vi "GageAcquire.vi"() -> ()   [LabVIEW 2015]
panel:
  in  "Force Capture":bool
  in  "Trigger":T1={"Slope"=0, "Level"=0, "Source"=0, "External Range"=2000, "External Coupling"=0, "External"=FALSE, "Disable"=FALSE, "External Impedance"=1} {"External Impedance" items=["50 Ohm", "HiZ"]; "External Coupling" items=["DC", "AC"]; "External Range" min=2000 max=10000 step=8000; "Slope" items=["Rising", "Falling"]; "Level" min=-100 max=100; "Source" min=0 max=64 step=1}
  in  "Channels":T2(array[cluster])=[{"Coupling"=0, "Differential Input"=FALSE, "Direct-to-ADC"=FALSE, "Range"=2000, "Impedance"=50, "DC Offset"=0, "Filter"=0}] {"Impedance" min=50 max=1000000 step=999950; "Coupling" items=["DC", "AC"]}
  in  "Acquisition":T3={"Sample Rate"=100000000.0, "Clock mode"=enum."Internal", "Mode"=0, "Depth"=8192.0, "Segment Size"=8192.0, "Trigger Timeout"=1000000.0, "Trigger Holdoff"=0.0, "Trigger Delay"=0.0} {"Segment Size" min=256.0 step=128.0; "Trigger Holdoff" min=0.0 step=128.0; "Trigger Delay" min=0.0 step=128.0; "Depth" min=256.0 step=128.0; "Mode" items=["Single", "Dual", "Quad", "Octal"]}
  in  "Continuous":bool
  out "Progress":string
  in  "stop":bool
  out "Waveform Graph":cluster{dbl, dbl, "Data in Volts":dbl[][]}(graph)
  out "System Name":string
  out "Sample Bits":i32
  out "Trigger Count":i32
  out "Channel Count":i32
  out "Board Count":i32
  out "System Count":i32
  in  "Points":u32=4096
  in  "Start":dbl
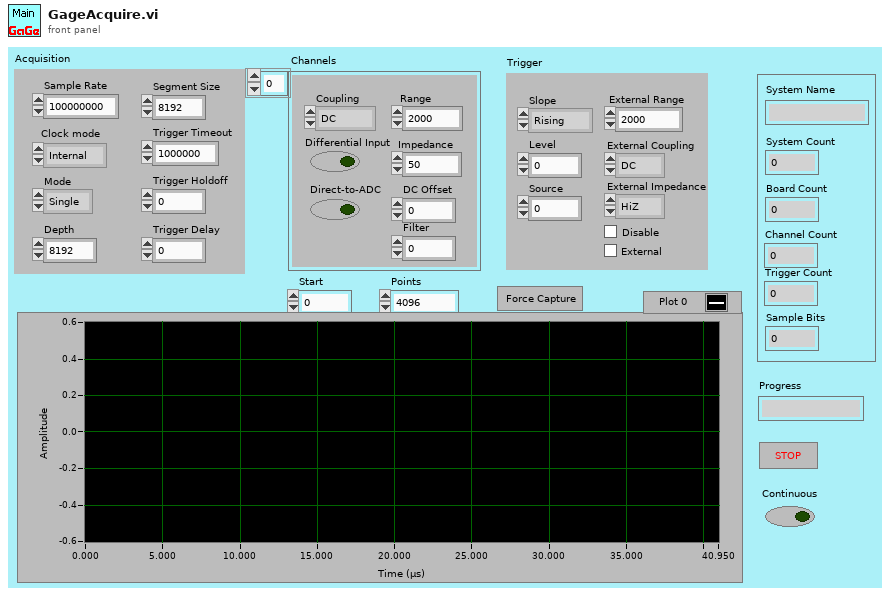
[diagram p1: front panel]
types:
  T1 = cluster{"Slope":u16, "Level":i32, "Source":i32, "External Range":u32, "External Coupling":u16, "External":bool, "Disable":bool, "External Impedance":u16}
  T2 = cluster{"Coupling":u16, "Differential Input":bool, "Direct-to-ADC":bool, "Range":u32, "Impedance":u32, "DC Offset":i32, "Filter":i32}[]
  T3 = cluster{"Sample Rate":dbl, "Clock mode":enum16{"Internal", "External", "Reference"}, "Mode":u16, "Depth":dbl, "Segment Size":dbl, "Trigger Timeout":dbl, "Trigger Holdoff":dbl, "Trigger Delay":dbl}
  T4 = cluster{"Handle":u32, "Sample size":u32, "Resolution":i32, "Offset":i32, "Channels":u32, "Boards":u32}
  T5 = cluster{"Coupling":u16, "Differential Input":bool, "Direct-to-ADC":bool, "Range":u32, "Impedance":u32, "DC Offset":i32, "Filter":i32}
  T6 = cluster{string, "Differential Input":bool, "Direct-to-ADC":bool, "Range":u32, "Impedance":u32, "DC Offset":i32, u32}
  T7 = cluster{"RingText.Text":string, "Level":i32, "Source":i32, "External Range":u32, "RingText.Text":string, "External":bool, "Disable":bool, "RingText.Text":string}
  T8 = cluster{"RingText.Text":string, "Level":i32, "Source":i32, "External Range":u32, "RingText.Text":string, "External":bool, "Disable":bool, "RingText.Text":string}[]
  T9 = cluster{"Sample Rate":dbl, "Clock mode":enum16{"Internal", "External", "Reference"}, "RingText.Text":string, "Depth":dbl, "Segment Size":dbl, "Trigger Timeout":dbl, "Trigger Holdoff":dbl, "Trigger Delay":dbl}
  T10 = cluster{"Handle":u32, "Sample Size":u32, "Resolution":i32, "Offset":i32, "Channels":u32, "Boards":u32}
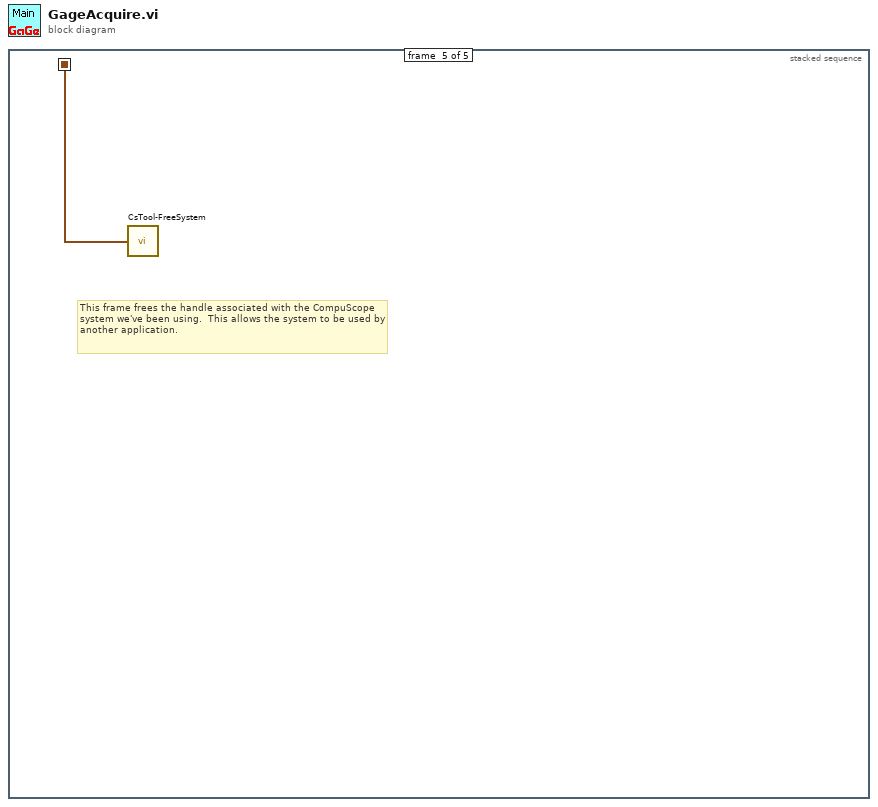
[diagram p0: block diagram]
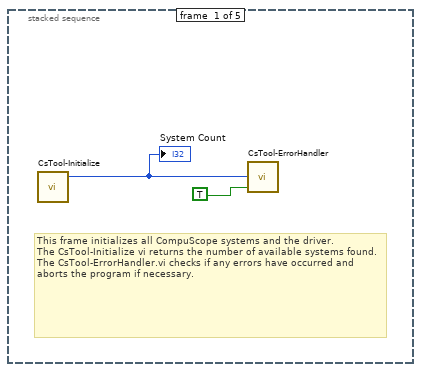
[diagram p2: hidden frame]
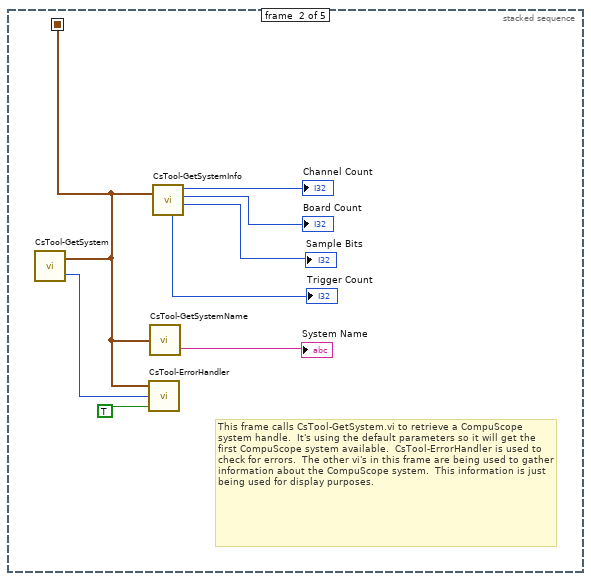
[diagram p3: hidden frame]
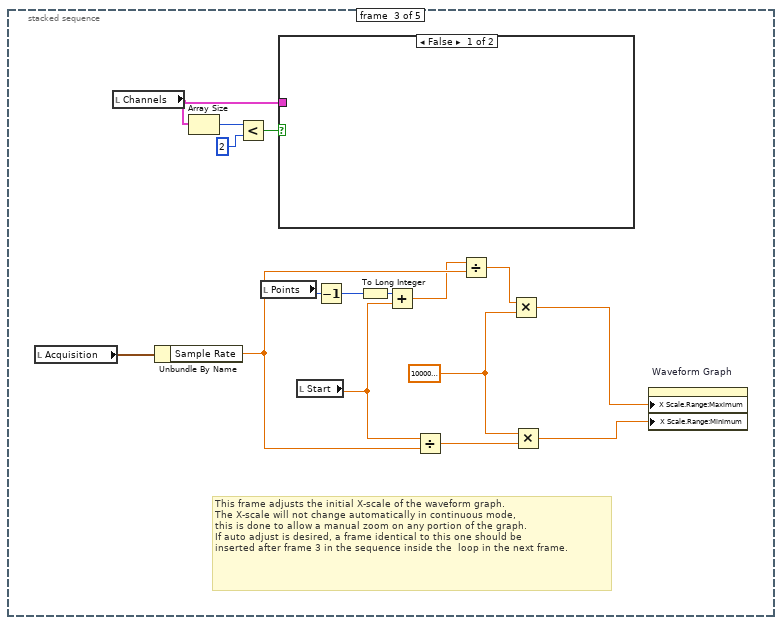
[diagram p4: hidden frame]
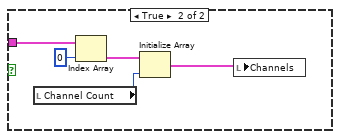
[diagram p5: hidden frame]
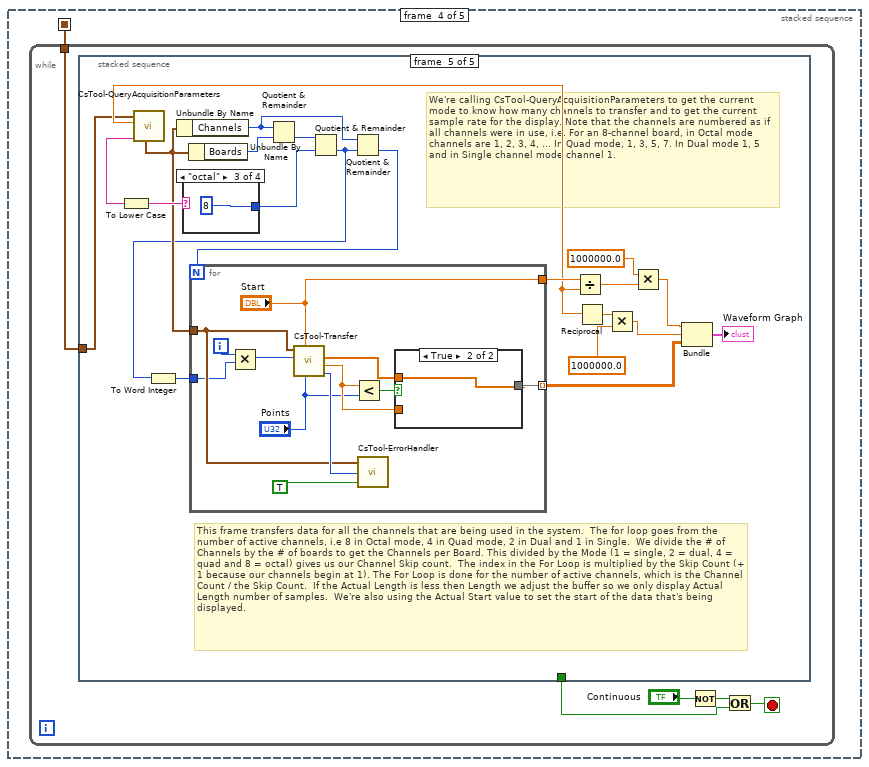
[diagram p6: hidden frame]
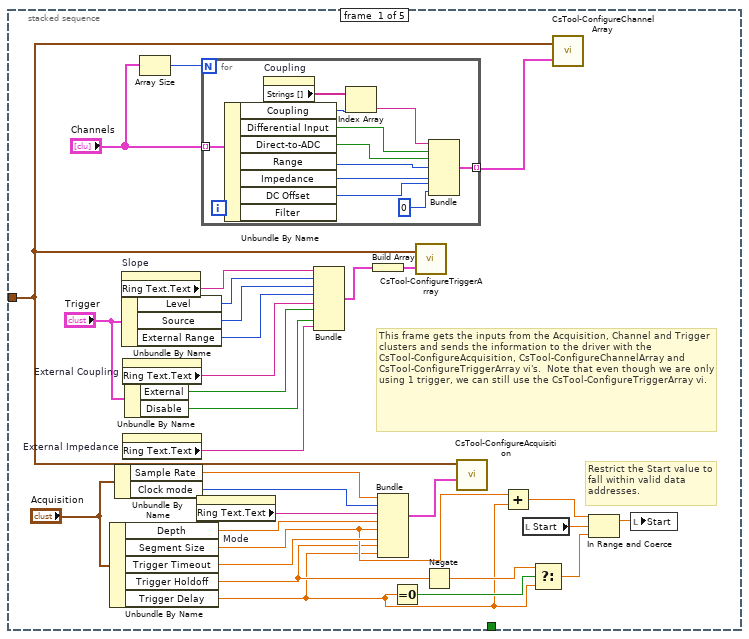
[diagram p7: hidden frame]
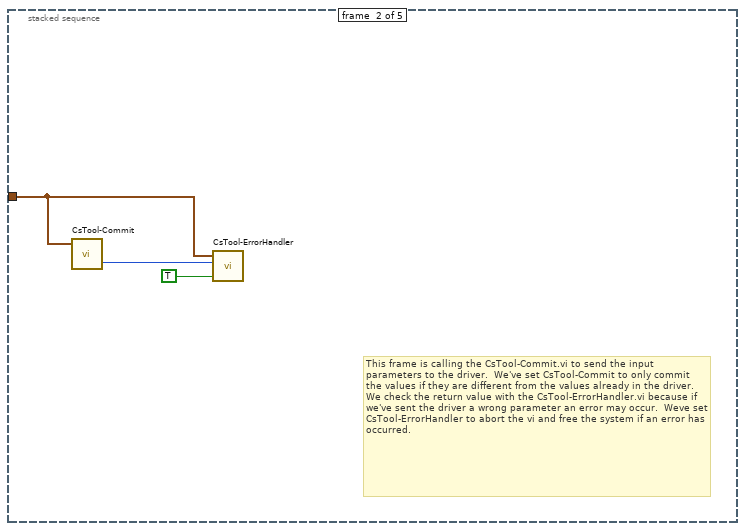
[diagram p8: hidden frame]
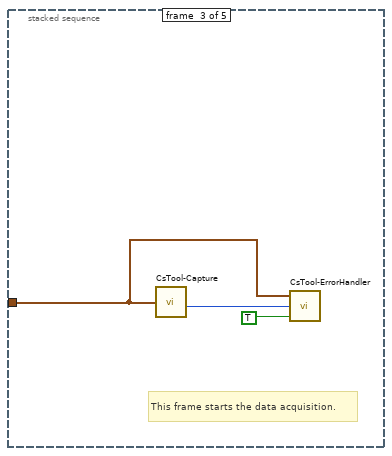
[diagram p9: hidden frame]
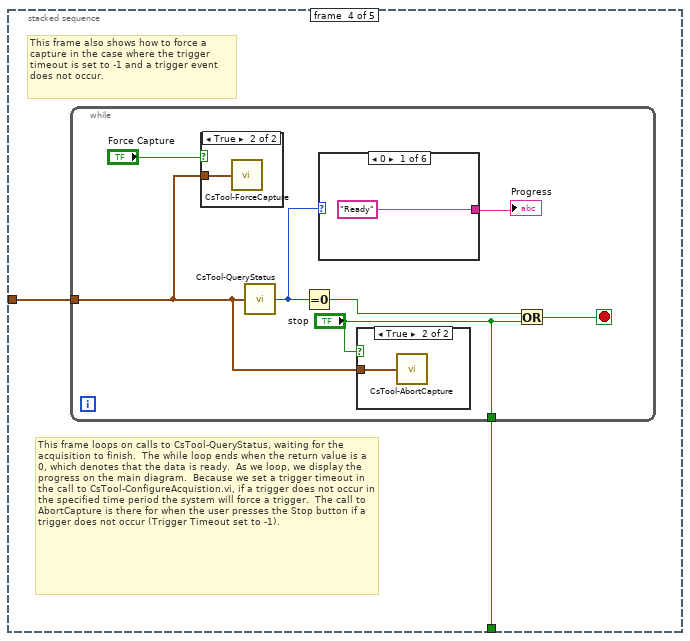
[diagram p10: hidden frame]
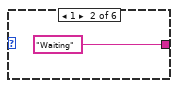
[diagram p13: hidden frame]
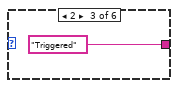
[diagram p14: hidden frame]
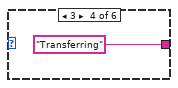
[diagram p15: hidden frame]
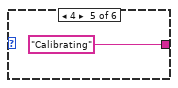
[diagram p16: hidden frame]
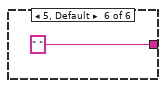
[diagram p17: hidden frame]
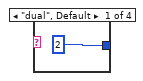
[diagram p18: hidden frame]
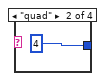
[diagram p19: hidden frame]
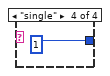
[diagram p20: hidden frame]
diagram:
  n1 = stacked-sequence {
    seq-local: [_ w5 _ _ _] -> [_ _ _ w32 w145]
    frame #0 {
      # "This frame initializes all CompuScope systems and the driver.\nThe CsTool-Initialize vi returns the number of available systems found.  The CsTool-ErrorHandler.vi checks if any errors have occurred and aborts the program if necessary."
      n2 = call <userlib>:"CsTool-Initialize.vi"() -> ("Number Of Systems"=w2:i32)  [unwired: 1 out]
      "System Count" <- w2
      n3 = call <userlib>:"CsTool-ErrorHandler.vi"("StopOnError (true)"=TRUE, "Error Code"=w2) -> ()  [unwired: 1 in, 1 out]
    }
    frame #1 {
      # "This frame calls CsTool-GetSystem.vi to retrieve a CompuScope system handle.  It's using the default parameters so it will get the first CompuScope system available.  CsTool-ErrorHandler is used to check for errors.  The other vi's in this frame are being used to gather information about the CompuScope system.  This information is just being used for display purposes."
      n4 = call <userlib>:"CsTool-GetSystem.vi"() -> ("Error Code"=w7:i32, "Handle Cluster"=w5:T4)  [unwired: 4 in]
      n5 = call <userlib>:"CsTool-ErrorHandler.vi"("StopOnError (true)"=TRUE, "Error Code"=w7, "Handle Cluster"=w5) -> ()  [unwired: 1 out]
      n6 = call <userlib>:"CsTool-GetSystemName.vi"("Handle Cluster"=w5) -> ("System Name"=→"System Name":string)  [unwired: 1 out]
      n7 = call <userlib>:"CsTool-GetSystemInfo.vi"("Handle Cluster"=w5) -> ("Number Of Triggers"=→"Trigger Count":u32, "Number Of Channels"=→"Channel Count":u32, "Number Of Boards"=→"Board Count":u32, "Sample Bits"=→"Sample Bits":u32)  [unwired: 3 out]
    }
    frame #2 {
      w17 = 1000000.0
      # "This frame adjusts the initial X-scale of the waveform graph.\nThe X-scale will not change automatically in continuous mode, \nthis is done to allow a manual zoom on any portion of the graph.\nIf auto adjust is desired, a frame identical to this one should be\ninserted after frame 3 in the sequence inside the  loop in the next frame."
      n8 = local read "Acquisition"() -> (w25:T3)
      n9 = local read "Channels"() -> (w15:T2)
      n10 = Unbundle By Name(w25) -> ("Sample Rate"=w24:dbl)
      n11 = Array Size(array=w15) -> (size(s)=w14:i32)
      n12 = Less?(x=w14, y=2) -> (x < y?=w16:bool)
      n13 = local read "Points"() -> (w23:u32)
      n14 = case shown="False" w16 {
        tunnel: w15 -> [_ w29]
        frame False {
        }
        frame True {
          n15 = local read "Channel Count"() -> (w31:i32)
          n16 = Index Array(array=w29, index=0) -> (element=w28:T5)
          n17 = Initialize Array(w28, w31) -> (w27:T2)
          n18 = local write "Channels"(w27) -> ()
        }
      }
      n19 = local read "Start"() -> (w22:dbl)
      n20 = Decrement(x=w23) -> (x-1=w11:u32)
      n21 = To Long Integer(number=w11) -> (32bit integer=w12:i32)
      n22 = Add(x=w12, y=w22) -> (x+y=w19:dbl)
      n23 = Divide(x=w22, y=w24) -> (x/y=w18:dbl)
      n24 = Divide(x=w19, y=w24) -> (x/y=w26:dbl)
      n25 = Multiply(x=w26, y=w17) -> (x*y=w21:dbl)
      n26 = Multiply(x=w17, y=w18) -> (x*y=w20:dbl)
      n27 = property on="Waveform Graph" class="WFGraph (strict)"("X Scale.Range:Maximum"=w21, "X Scale.Range:Minimum"=w20) -> ()  [unwired: 2 in, 2 out]
    }
    frame #3 {
      n28 = while {
        tunnel: w32 -> [w37]
        stop <- w34 stop-if-true
        n29 = stacked-sequence {
          tunnel: w37 -> [w57 w80 w83 w87 w114]
          tunnel: [_ _ _ w86 _] -> w33
          frame #0 {
            # "Restrict the Start value to fall within valid data addresses."
            # "This frame gets the inputs from the Acquisition, Channel and Trigger clusters and sends the information to the driver with the CsTool-ConfigureAcquisition, CsTool-ConfigureChannelArray and CsTool-ConfigureTriggerArray vi's.  Note that even though we are only using 1 trigger, we can still use the CsTool-ConfigureTriggerArray vi."
            n30 = Unbundle By Name("Acquisition") -> ("Depth"=w62:dbl, "Segment Size"=w46:dbl, "Trigger Timeout"=w52:dbl, "Trigger Holdoff"=w45:dbl, "Trigger Delay"=w42:dbl)
            n31 = Unbundle By Name("Acquisition") -> ("Sample Rate"=w64:dbl, "Clock mode"=w53:enum16{"Internal", "External", "Reference"})
            n32 = property on="Slope" class="Ring (strict)"() -> ("Ring Text.Text"=w68:string)  [unwired: 2 in, 2 out]
            n33 = Unbundle By Name("Trigger") -> ("Level"=w67:i32, "Source"=w50:i32, "External Range"=w49:u32)
            n34 = property on="External Coupling" class="Ring (strict)"() -> ("Ring Text.Text"=w66:string)  [unwired: 2 in, 2 out]
            n35 = property on="External Impedance" class="Ring (strict)"() -> ("Ring Text.Text"=w47:string)  [unwired: 2 in, 2 out]
            n36 = Unbundle By Name("Trigger") -> ("External"=w54:bool, "Disable"=w48:bool)
            n37 = Array Size(array="Channels") -> (size(s)=w60:i32)
            n38 = property on="Mode" class="Ring (strict)"() -> ("Ring Text.Text"=w63:string)  [unwired: 2 in, 2 out]
            n39 = for {
              N: w60 -> [_]
              tunnel: "Channels" -> [w77] mode=indexing
              tunnel: [w78] -> w59 mode=indexing
              n40 = Unbundle By Name(w77) -> ("Coupling"=w73:u16, "Differential Input"=w79:bool, "Direct-to-ADC"=w72:bool, "Range"=w71:u32, "Impedance"=w70:u32, "DC Offset"=w69:i32)  [unwired: 1 out]
              n41 = property on="Coupling" class="Ring (strict)"() -> ("Strings []"=w76:string[])  [unwired: 2 in, 2 out]
              n42 = Index Array(array=w76, index=w73) -> (element=w75:string)
              n43 = Bundle(w75, "Differential Input"=w79, "Direct-to-ADC"=w72, "Range"=w71, "Impedance"=w70, "DC Offset"=w69, u32 0) -> (w78:T6)  [unwired: 1 in]
            }
            n44 = Bundle("RingText.Text"=w68, "Level"=w67, "Source"=w50, "External Range"=w49, "RingText.Text"=w66, "External"=w54, "Disable"=w48, "RingText.Text"=w47) -> (w65:T7)  [unwired: 1 in]
            n45 = Build Array(w65) -> (w56:T8)
            n46 = Bundle("Sample Rate"=w64, "Clock mode"=w53, "RingText.Text"=w63, "Depth"=w62, "Segment Size"=w46, "Trigger Timeout"=w52, "Trigger Holdoff"=w45, "Trigger Delay"=w42) -> (w51:T9)  [unwired: 1 in]
            n47 = Equal To 0?(x=w42) -> (x = 0?=w44:bool)
            n48 = call <userlib>:"CsTool-ConfigureTriggerArray.vi"("Triggers"=w56, "Handle Cluster"=w57) -> ()  [unwired: 1 out]
            n49 = Negate(x=w45) -> (-x=w43:dbl)
            n50 = call <userlib>:"CsTool-ConfigureAcquisition.vi"("Handle Cluster"=w57, "Acquisition"=w51) -> ()  [unwired: 3 in, 1 out]
            n51 = Add(x=w46, y=w42) -> (x+y=w40:dbl)
            n52 = local read "Start"() -> (w39:dbl)
            n53 = Select(t=w43, s=w44, f=w42) -> (s? t:f=w41:dbl)
            n54 = call <userlib>:"CsTool-ConfigureChannelArray.vi"("Channels"=w59, "Handle Cluster"=w57) -> ()  [unwired: 1 out]
            n55 = In Range and Coerce(upper limit=w40, x=w39, lower limit=w41) -> (coerced(x)=w38:dbl)  [unwired: 1 out]
            n56 = local write "Start"(w38) -> ()
          }
          frame #1 {
            # "This frame is calling the CsTool-Commit.vi to send the input parameters to the driver.  We've set CsTool-Commit to only commit the values if they are different from the values already in the driver.  We check the return value with the CsTool-ErrorHandler.vi because if we've sent the driver a wrong parameter an error may occur.  Weve set CsTool-ErrorHandler to abort the vi and free the system if an error has occurred."
            n57 = call <userlib>:"CsTool-Commit.vi"("Handle Cluster"=w80) -> ("Error Code"=w82:i32)  [unwired: 2 in, 1 out]
            n58 = call <userlib>:"CsTool-ErrorHandler.vi"("StopOnError (true)"=TRUE, "Error Code"=w82, "Handle Cluster"=w80) -> ()  [unwired: 1 out]
          }
          frame #2 {
            # "This frame starts the data acquisition."
            n59 = call <userlib>:"CsTool-Capture.vi"("Handle Cluster"=w83) -> ("Error Code"=w85:i32)
            n60 = call <userlib>:"CsTool-ErrorHandler.vi"("StopOnError (true)"=TRUE, "Error Code"=w85, "Handle Cluster"=w83) -> ()  [unwired: 1 out]
          }
          frame #3 {
            # "This frame also shows how to force a capture in the case where the trigger timeout is set to -1 and a trigger event does not occur."
            # "This frame loops on calls to CsTool-QueryStatus, waiting for the acquisition to finish.  The while loop ends when the return value is a 0, which denotes that the data is ready.  As we loop, we display the progress on the main diagram.  Because we set a trigger timeout in the call to CsTool-ConfigureAcquistion.vi, if a trigger does not occur in the specified time period the system will force a trigger.  The call to AbortCapture is there for when the user presses the Stop button if a trigger does not occur (Trigger Timeout set to -1)."
            n61 = while {
              tunnel: w87 -> [w88]
              tunnel: ["stop"] -> w86
              stop <- w91 stop-if-true
              n62 = case shown="True" "Force Capture" {
                tunnel: w88 -> [_ w95]
                frame False {
                }
                frame True {
                  n63 = call <userlib>:"CsTool-ForceCapture.vi"("Handle Cluster"=w95) -> ()  [unwired: 1 out]
                }
              }
              n64 = call <userlib>:"CsTool-QueryStatus.vi"("Handle Cluster"=w88) -> ("Status"=w94:i32)
              n65 = Equal To 0?(x=w94) -> (x = 0?=w92:bool)
              n66 = case shown="0" w94 {
                tunnel: ["Ready" "Waiting" "Triggered" "Transferring" "Calibrating" " "] -> w93
                frame 0 {
                }
                frame 1 {
                }
                frame 2 {
                }
                frame 3 {
                }
                frame 4 {
                }
                frame 5, Default {
                }
              }
              "Progress" <- w93
              n67 = case shown="True" "stop" {
                tunnel: w88 -> [_ w96]
                frame False {
                }
                frame True {
                  n68 = call <userlib>:"CsTool-AbortCapture.vi"("Handle Cluster"=w96) -> ()  [unwired: 1 out]
                }
              }
              n69 = Or(x=w92, y="stop") -> (x .or. y?=w91:bool)
            }
          }
          frame #4 {
            # "We're calling CsTool-QueryAcquisitionParameters to get the current mode to know how many channels to transfer and to get the current sample rate for the display. Note that the channels are numbered as if all channels were in use, i.e. For an 8-channel board, in Octal mode channels are 1, 2, 3, 4, ... In Quad mode, 1, 3, 5, 7. In Dual mode 1, 5 and in Single channel mode channel 1."
            # "This frame transfers data for all the channels that are being used in the system.  The for loop goes from the number of active channels, i.e 8 in Octal mode, 4 in Quad mode, 2 in Dual and 1 in Single.  We divide the # of Channels by the # of boards to get the Channels per Board. This divided by the Mode (1 = single, 2 = dual, 4 = quad and 8 = octal) gives us our Channel Skip count.  The index in the For Loop is multiplied by the Skip Count (+ 1 because our channels begin at 1). The For Loop is done for the number of active channels, which is the Channel Count / the Skip Count.  If the Actual Length is less then Length we adjust the buffer so we only display Actual Length number of samples.  We're also using the Actual Start value to set the start of the data that's being displayed."
            n70 = call <userlib>:"CsTool-QueryAcquisitionParameters.vi"("Handle Cluster"=w114) -> ("Output Handle Cluster"=w110:T10, "Mode"=w113:string, "Sample Rate"=w115:dbl)  [unwired: 8 out]
            n71 = To Lower Case(string=w113) -> (all lower case string=w112:string)
            n72 = Unbundle By Name(w110) -> ("Channels"=w107:u32)
            n73 = case shown="\"octal\"" w112 {
              tunnel: [2 4 8 1] -> w106
              frame "dual", Default {
              }
              frame "quad" {
              }
              frame "octal" {
              }
              frame "single" {
              }
            }
            n74 = Unbundle By Name(w110) -> ("Boards"=w109:u32)
            n75 = Quotient & Remainder(x=w107, y=w109) -> (floor(x/y)=w108:u32)  [unwired: 1 out]
            n76 = Quotient & Remainder(x=w108, y=w106) -> (floor(x/y)=w105:u32)  [unwired: 1 out]
            n77 = To Word Integer(number=w105) -> (16bit integer=w111:i16)
            n78 = Quotient & Remainder(x=w107, y=w105) -> (floor(x/y)=w104:u32)  [unwired: 1 out]
            n79 = for {
              N: w104 -> [_]
              tunnel: ["Start"] -> w119
              tunnel: [w136] -> w118 mode=indexing
              tunnel: w110 -> [w133]
              tunnel: w111 -> [w130]
              i -> [w131]
              n80 = Multiply(x=w131, y=w130) -> (x*y=w129:i32)
              n81 = call <userlib>:"CsTool-Transfer.vi"("Length (4096)"="Points", "Start (0)"="Start", "Channel (0)"=w129, "Handle Cluster"=w133) -> ("Error Code"=w135:i32, "Actual Length"=w138:dbl, "Data in Volts"=w137:dbl[])  [unwired: 2 in, 1 out]
              n82 = Less?(x=w138, y="Points") -> (x < y?=w139:bool)
              n83 = call <userlib>:"CsTool-ErrorHandler.vi"("StopOnError (true)"=TRUE, "Error Code"=w135, "Handle Cluster"=w133) -> ()  [unwired: 1 out]
              n84 = case shown="True" w139 {
                tunnel: w137 -> [w143 w144]
                tunnel: w138 -> [w141 _]
                tunnel: [w140 w144] -> w136
                frame False {
                  n85 = Array Subset(array=w143, index=0, length=w141) -> (w140:dbl[])
                }
                frame True {
                }
              }
            }
            n86 = Divide(x=w119, y=w115) -> (x/y=w123:dbl)
            n87 = Reciprocal(x=w115) -> (1/x=w120:dbl)
            n88 = Multiply(x=w120, y=1000000.0) -> (x*y=w122:dbl)
            n89 = Multiply(x=1000000.0, y=w123) -> (x*y=w103:dbl)
            n90 = Bundle(w103, w122, "Data in Volts"=w118) -> (→"Waveform Graph":cluster{dbl, dbl, "Data in Volts":dbl[][]})  [unwired: 1 in]
          }
        }
        n91 = Not(x="Continuous") -> (.not. x?=w36:bool)
        n92 = Or(x=w36, y=w33) -> (x .or. y?=w34:bool)
      }
    }
    frame #4 {
      # "This frame frees the handle associated with the CompuScope system we've been using.  This allows the system to be used by another application."
      n93 = call <userlib>:"CsTool-FreeSystem.vi"("Handle Cluster"=w145) -> ()  [unwired: 1 out]
    }
  }
